vi "testPhasePlotting_modulo_useCustomVI.vi"() -> ()   [LabVIEW 2025]
uses:
  <vilib>/measure/NI_MAPro.lvlib
panel:
  out "Phase Waveform":waveform(dbl)(graph)
  in  "Sampling info":cluster{"Fs":dbl, "#s":dbl}={"Fs"=10000.0, "#s"=1000.0} {"Fs" format="%.2p"}
  out "Frequency waveform":dynamicdata(graph)
  in  "stop":bool
  in  "Phase Unit":u16(ring) items=["Degree", "Radian"]
  out "Nominal Frequency unit (Hz)":string="Hz"
  out "Frequency unit (Hz)":string="Hz"
  out "Phase unit (deg)":string="deg"
  out "Phase  unit (rad)":string="rad"
  in  "Nominal Frequency":dbl=50.0
  in  "Frequency":dbl=50.0
  in  "Phase":dbl
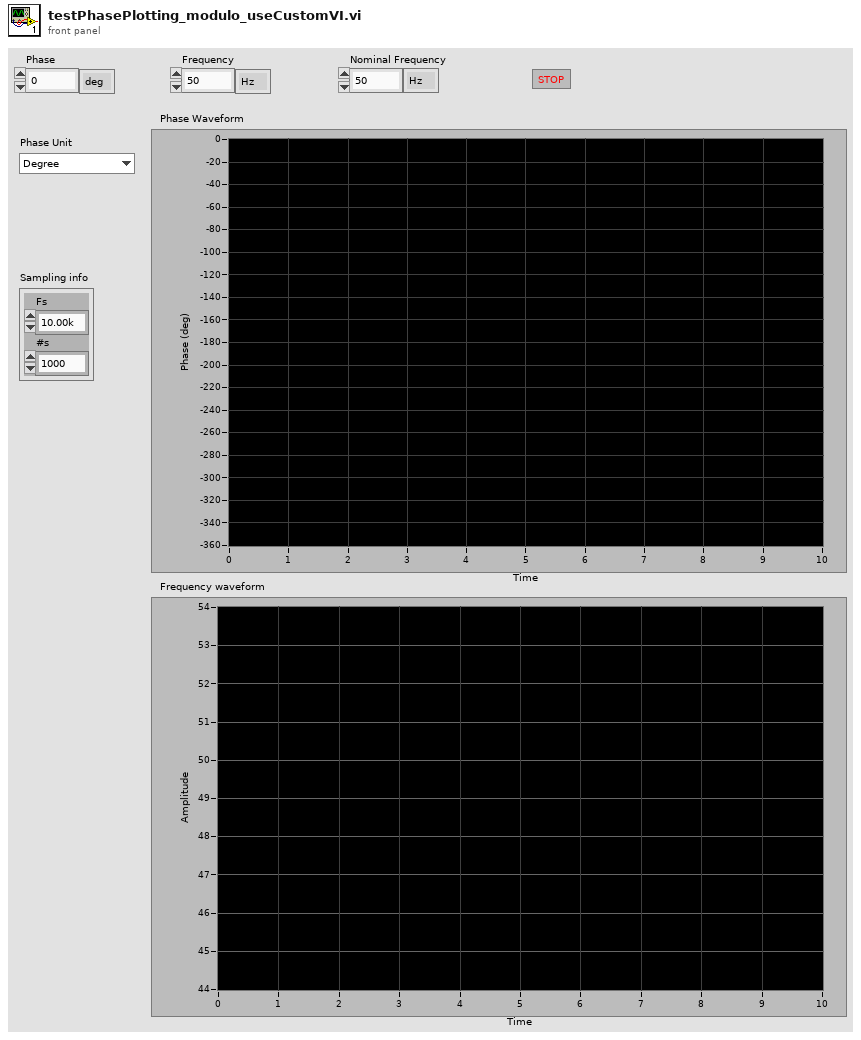
[diagram p1: front panel]
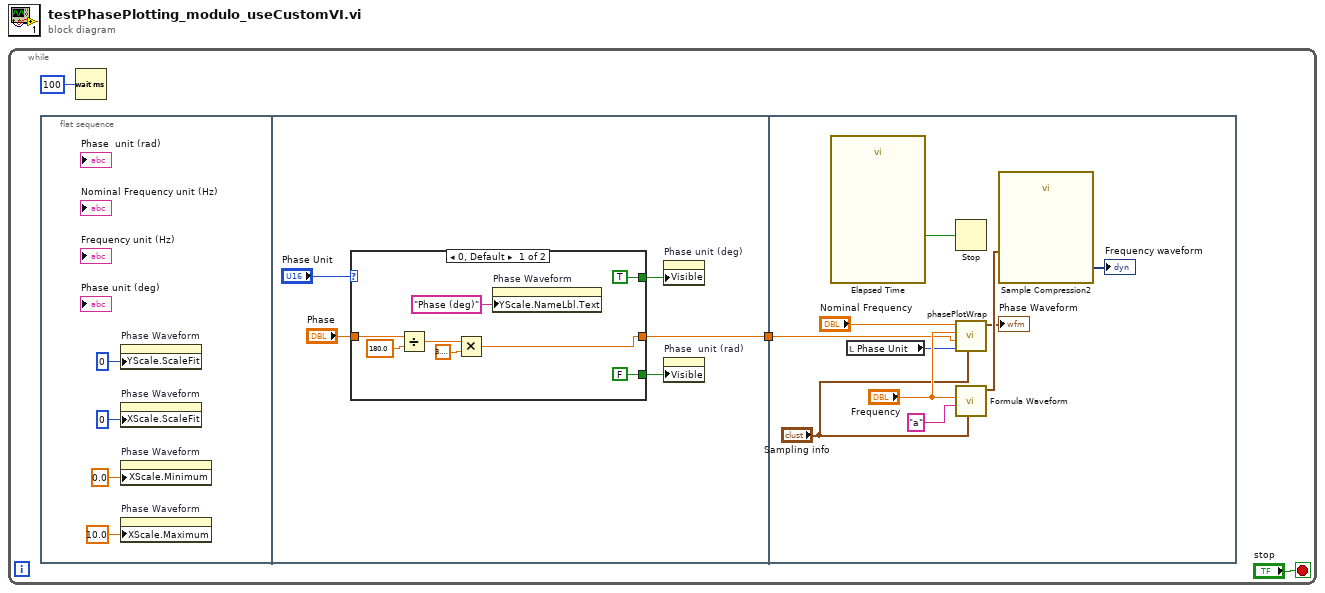
[diagram p0: block diagram]
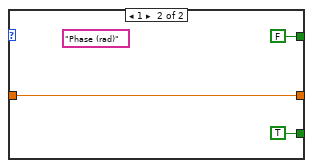
[diagram p2: hidden frame]
diagram:
  n1 = while {
    stop <- "stop" stop-if-true
    n2 = flat-sequence {
      tunnel: [w9] -> w3
      tunnel: w3 -> [w27]
      frame #0 {
        n3 = property on="Phase Waveform" class="WFChart (strict)"("YScale.ScaleFit"=u8 0 ("Y Scale.Scale Fit")) -> ()  [unwired: 2 in, 2 out]
        n4 = property on="Phase Waveform" class="WFChart (strict)"("XScale.ScaleFit"=u8 0 ("X Scale.Scale Fit")) -> ()  [unwired: 2 in, 2 out]
        n5 = property on="Phase Waveform" class="WFChart (strict)"("XScale.Minimum"=0.0 ("X Scale.Range:Minimum")) -> ()  [unwired: 2 in, 2 out]
        n6 = property on="Phase Waveform" class="WFChart (strict)"("XScale.Maximum"=10.0 ("X Scale.Range:Maximum")) -> ()  [unwired: 2 in, 2 out]
      }
      frame #1 {
        n7 = case shown="0, Default" "Phase Unit" {
          tunnel: [TRUE FALSE] -> w12
          tunnel: [FALSE TRUE] -> w11
          tunnel: "Phase" -> [w17 w21]
          tunnel: [w14 w21] -> w9
          frame 0, Default {
            n8 = Divide(x=w17, y=180.0) -> (x/y=w16:dbl)
            n9 = Multiply(x=w16, y=3.141592653589793) -> (x*y=w14:dbl)
            n10 = property on="Phase Waveform" class="WFChart (strict)"("YScale.NameLbl.Text"="Phase (deg)" ("Y Scale.Name Label.Text")) -> ()  [unwired: 2 in, 2 out]
          }
          frame 1 {
            (unwired) "Phase (rad)" ("Y Scale.Name Label.Text")
          }
        }
        n11 = property on="Phase unit (deg)" class="Str"("Visible"=w12) -> ()  [unwired: 2 in, 2 out]
        n12 = property on="Phase  unit (rad)" class="Str"("Visible"=w11) -> ()  [unwired: 2 in, 2 out]
      }
      frame #2 {
        n13 = call "Elapsed Time"() -> ("Time has Elapsed"=w30:bool)  [unwired: 12 in, 7 out]
        n14 = local read "Phase Unit"() -> (w25:u16)
        n15 = Stop(stop? (T)=w30) -> ()
        n16 = call "phasePlotWrap.vi"("Sampling info"="Sampling info", "Phase Unit"=w25, "Phase"=w27, "Frequency"="Frequency", "Nominal Frequency"="Nominal Frequency") -> ("Phase waveform"=→"Phase Waveform":waveform(dbl))  [unwired: 6 in]
        n17 = call <vilib>:"Formula Waveform.vi"("sampling info"="Sampling info", "formula"="a", "amplitude"="Frequency") -> ("signal out"=w31:waveform(dbl))  [unwired: 7 in, 1 out]
        n18 = call "Sample Compression2"("Signals"=w31) -> ("Maximum"=→"Frequency waveform":dynamicdata)  [unwired: 8 in, 2 out]
      }
    }
    n19 = Wait (ms)(milliseconds to wait=u32 100) -> ()  [unwired: 1 out]
  }
